vi "Wrapper_getWavelengths.vi"(2 "Index":i32, 3 "Wrapper":u32) -> (0 "Length":i32, 1 "WL Values":dbl[](array[numeric]))   [LabVIEW 2012]
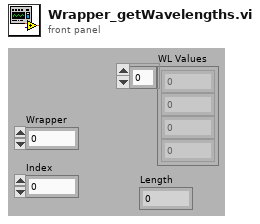
[diagram p1: front panel]
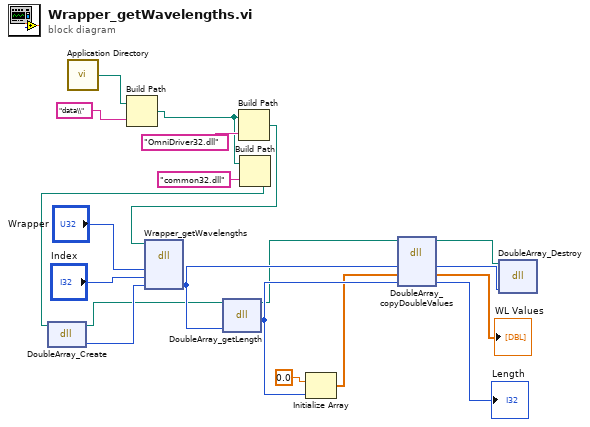
[diagram p0: block diagram]
diagram:
  n1 = call <vilib>:"Application Directory.vi"() -> ("Application Directory"=w10:path)
  n2 = Build Path(base path=w10, name or relative path="data\\") -> (appended path=w5:path)
  n3 = Build Path(base path=w5, name or relative path="OmniDriver32.dll") -> (appended path=w6:path)
  n4 = Build Path(base path=w5, name or relative path="common32.dll") -> (appended path=w1:path)
  n5 = dll-call lib="common32.dll" fn="DoubleArray_Create" label="DoubleArray.Create"(path in=w1) -> (path out=w4:path, "return type"=w18:u32)  [unwired: 2 in, 1 out]
  n6 = dll-call lib="D:/Software Development/EPI Development/BurnIn Testing/Instruments/Drivers/Ocean Optics/OOI_HOME/OmniDriver32.dll" fn="Wrapper_getWavelengths" label="Wrapper.getWavelengths"(path in=w6, "Wrapper"="Wrapper", "Index"="Index", "WL DoubleArray"=w18) -> ("WL DoubleArray"=w14:u32)  [unwired: 4 in, 3 out]
  n7 = dll-call lib="common32.dll" fn="DoubleArray_getLength" label="DoubleArray.getLength"(path in=w4, "DoubbleArray"=w14) -> (path out=w3:path, "return type"=w16:i32)  [unwired: 3 in, 1 out]
  n8 = Initialize Array(0.0 ("element"), w16) -> (w15:dbl[])
  n9 = dll-call lib="common32.dll" fn="DoubleArray_copyDoubleValues" label="DoubleArray.coopyDoubleValues"(path in=w3, "DoubleArray"=w14, "Values"=w15, "Length"=w16) -> (path out=w2:path, "DoubleArray"=w11:u32, "Values"=→"WL Values":dbl[], "Length"=→"Length":i32)  [unwired: 2 in, 2 out]
  n10 = dll-call lib="common32.dll" fn="DoubleArray_Destroy" label="DoubleArray.Destroy"(path in=w2, "DoubleArray"=w11) -> ()  [unwired: 3 in, 3 out]
